vi "_fgv_debug.vi"(7 "Operation":T1=enum."ReadCommand", 8 "error in":errorcluster caption="error in (no error)", 9 "Command in":string, 11 "VISA resource name":refnum<visa-resource-name>) -> (0 "error out":errorcluster, 3 "VISA resource name out":refnum<visa-resource-name>)   [LabVIEW 2022 SP3, in "hmp4000_rsidr_core.lvlib"]
uses:
  hmp4000_rsidr_core.lvlib
  _type_Operation_Fgv_Debug.ctl
  type_Error_Codes.ctl
  Trim Whitespace One-Sided.vi
  Match Regular Expression.xnode
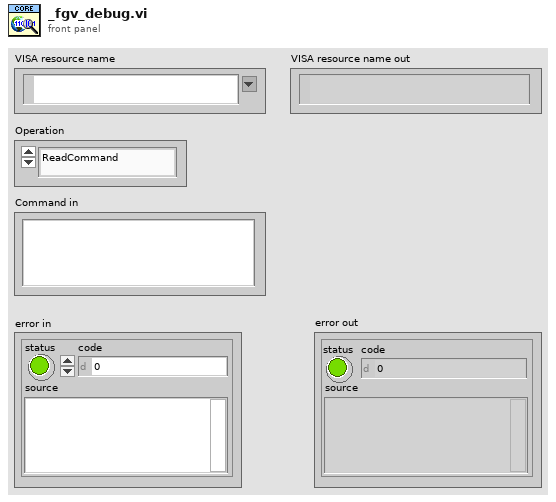
[diagram p1: front panel]
types:
  T1 = typedef "hmp4000_rsidr_core.lvlib/_type_Operation_Fgv_Debug.ctl" = enum16{"Reset", "ReadCommand", "SetCommand"}
  T2 = typedef "hmp4000_rsidr_core.lvlib/type_Error_Codes.ctl" = enum16{"No_error", "VISA_err_ResourceNotFound", "VISA_err_Timeout", "VISA_warn_MoreDataAvailable", "RS_err_MissingCallback", "RS_err_InvalidAttribute", "RS_err_InvalidValue", "RS_err_UnknownResource", "RS_err_AlreadyInitialized", "RS_err_InstrumentStatus", "RS_err_BadRepCapName", "RS_err_TypesMismatch", "RS_err_ValueNotSupported", "RS_err_InvalidRngTable", "RS_err_IDqueryFail", "RS_err_UnexpResponse", "VISA_warn_ConfigNotLoaded", "RS_err_AttributeNotReadable", "RS_err_AttributeNotWritable", "RS_err_InstrumentType", "RS_err_InstrumentOption", "VISA_err_InvalidSize", "RS_err_ReliabilityIndicator", "VISA_warn_UnknownStatus", "VISA_warn_TermCharRead", "VISA_err_IO_error", "RS_err_FunctionNotSupported", "VISA_warn_QueueEmpty"}
  T3 = typedef "hmp4000_rsidr_core.lvlib/type_Session_Data.ctl" = cluster{"IDN string":string, "Instrument FW":string, "Instr type":string, "Instr type for err. msg.":string, "Installed Options":string[], "Ignore Error Messages":string, "Logging params":variant, "OPC Timeout":i32, "VISA Timeout":i32, "STB Poll VISA Timeout":i32, "Additional Flags":i32, "Wait Before Read":i32, "Wait Before Write":i32, "Option String Flags":i32, "IO Segment Size":i64, "VISA Access Mode":T4, "Interface Type":T5, "OPC Wait Mode":T6, "Bin Float Number  Format":T7, "Bin Integer Number Format":T8, "Simulate":bool, "VXIcapable":bool, "Duplicate Session":bool, "Add LF to Write":bool, "Logging":bool, "Fast Sweep":bool, "Query Instrument Status":bool, "Check Range":bool, "Check Options":bool}
  T4 = typedef "hmp4000_rsidr_core.lvlib/type_VisaAccessMode.ctl" = u16
  T5 = typedef "hmp4000_rsidr_core.lvlib/type_InterfaceType.ctl" = enum16{"Unknown", "GPIB", "VXI", "GPIB_VXI", "ASRL", "PXI", "TCPIP", "USB", "SOCKET"}
  T6 = typedef "hmp4000_rsidr_core.lvlib/type_OPC_Wait_Mode.ctl" = enum16{"STBpolling", "STBpollingSlow", "STBpollingSuperSlow", "ServiceRequest", "OPCquery"}
  T7 = typedef "hmp4000_rsidr_core.lvlib/type_Binary_Float_Number_Format.ctl" = enum16{"Float_4_Bytes_Swapped", "Float_4_Bytes", "Double_8_Bytes_Swapped", "Double_8_Bytes"}
  T8 = typedef "hmp4000_rsidr_core.lvlib/type_Binary_Integer_Number_Format.ctl" = enum16{"Int32_4_Bytes_Swapped", "Int32_4 Bytes", "Int16_2_Bytes_Swapped", "Int16_2_Bytes"}
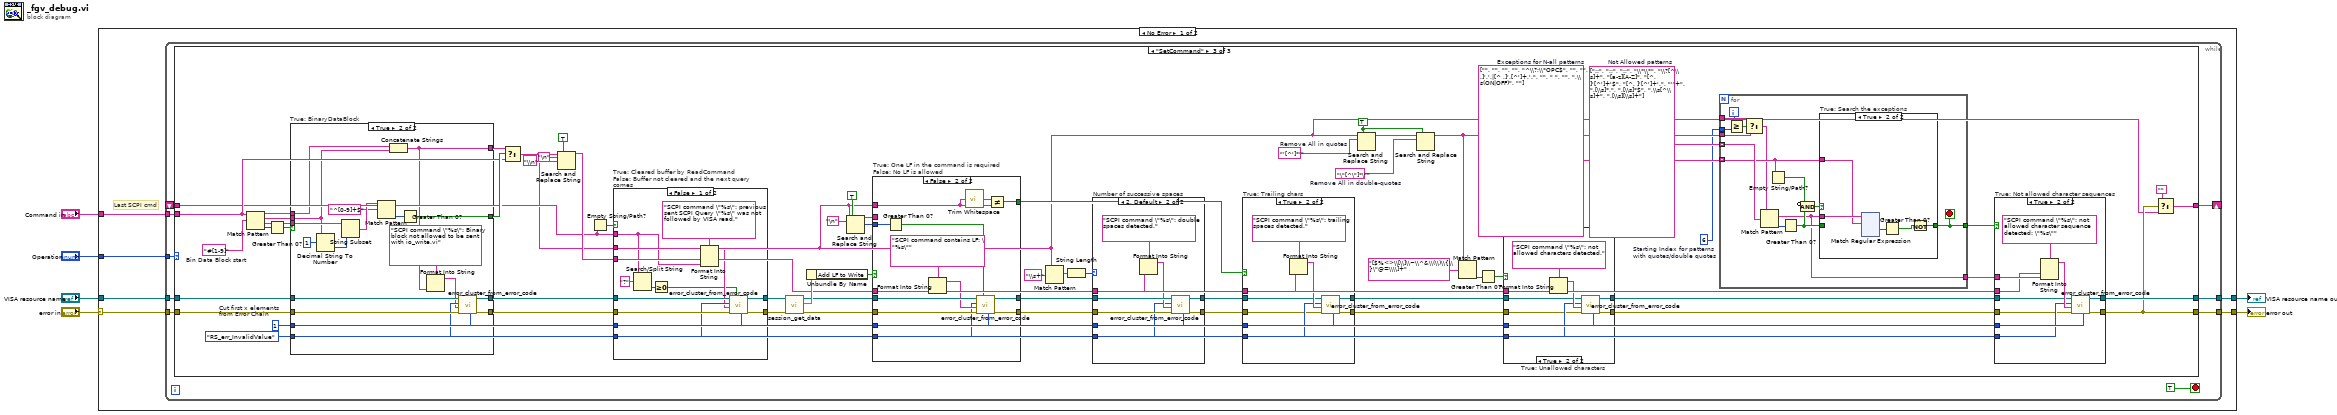
[diagram p0: block diagram]
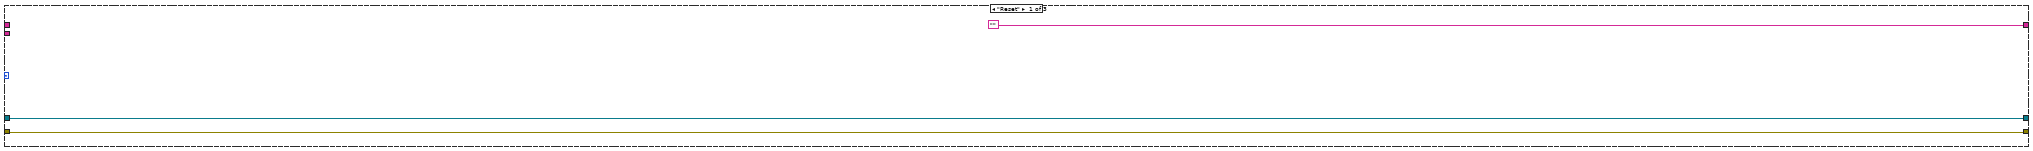
[diagram p2: hidden frame]
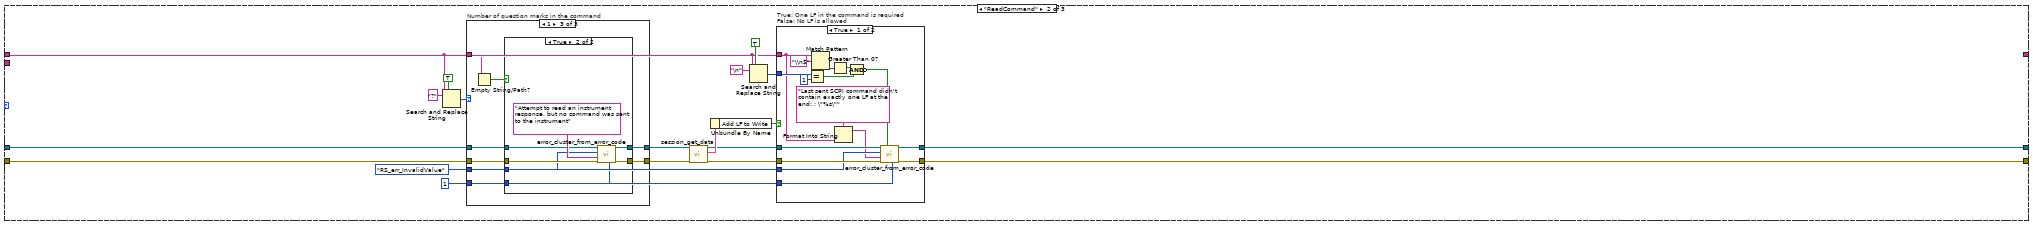
[diagram p3: hidden frame]
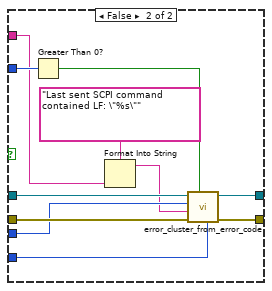
[diagram p4: hidden frame]
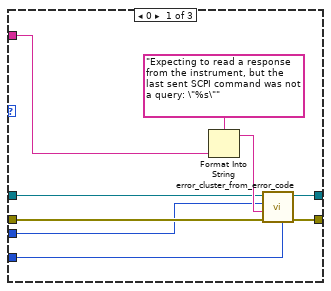
[diagram p5: hidden frame]
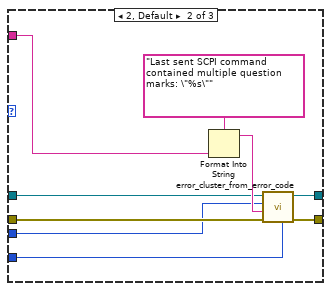
[diagram p6: hidden frame]
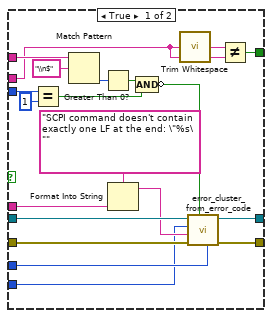
[diagram p13: hidden frame]
diagram:
  n1 = case shown="No Error" "error in" {
    selector: "error in" -> [w8 w420]
    tunnel: [w10 w420] -> w2
    tunnel: "Operation" -> [w12 _]
    tunnel: "Command in" -> [w11 _]
    tunnel: "VISA resource name" -> [w7 w419]
    tunnel: [w9 w419] -> w1
    frame No Error {
      # "Last SCPI cmd"
      n2 = while {
        shift-right: [w18] -> _
        shift-left: _ -> [w17]
        tunnel: w12 -> [w20]
        tunnel: w8 -> [w14]
        tunnel: w11 -> [w19]
        tunnel: w7 -> [w13]
        tunnel: [w16] -> w10
        tunnel: [w15] -> w9
        stop <- TRUE stop-if-true
        n3 = case shown="\"SetCommand\"" w20 {
          tunnel: w19 -> [_ _ w126]
          tunnel: ["" ("Empty String Constant") _ w161] -> w18
          tunnel: w17 -> [_ w28 w125]
          tunnel: w14 -> [w23 w40 w111]
          tunnel: w13 -> [w22 w39 w110]
          tunnel: [w23 w27 w140] -> w16
          tunnel: [w22 w26 w141] -> w15
          frame "Reset" {
          }
          frame "ReadCommand" {
            w25 = 1 ("Cut first x elements\nfrom Error Chain (0)")
            w31 = type_Error_Codes."RS_err_InvalidValue" ("Error Enum in")
            n4 = Search and Replace String(replace all?=TRUE ("replace all? (F)"), input string=w28, search string="?") -> (number of replacements=w41:i32)  [unwired: 5 in, 3 out]
            n5 = case "Number of question marks in the command" shown="1" w41 {
              tunnel: w40 -> [w78 w87 w94]
              tunnel: [w77 w86 w92] -> w38
              tunnel: w28 -> [w76 w85 w96]
              tunnel: w39 -> [w74 w82 w93]
              tunnel: [w73 w84 w91] -> w37
              tunnel: w31 -> [w72 w81 w90]
              tunnel: w25 -> [w71 w80 w89]
              frame 0 {
                n6 = Format Into String(format string="Expecting to read a response from the instrument, but the last sent SCPI command was not a query: \"%s\"", w76) -> (resulting string=w75:string)  [unwired: 2 in, 1 out]
                n7 = call "error_cluster_from_error_code.vi"("Cut first x elements\nfrom Error Chain (0)"=w71, "error in"=w78, "Error Message (\"\")"=w75, "Error Enum in"=w72, "VISA resource name"=w74) -> ("error out"=w77:errorcluster, "VISA resource name out"=w73:refnum<visa-resource-name>)  [unwired: 5 in]
              }
              frame 2, Default {
                n8 = Format Into String(format string="Last sent SCPI command contained multiple question marks: \"%s\"", w85) -> (resulting string=w83:string)  [unwired: 2 in, 1 out]
                n9 = call "error_cluster_from_error_code.vi"("Cut first x elements\nfrom Error Chain (0)"=w80, "error in"=w87, "Error Message (\"\")"=w83, "Error Enum in"=w81, "VISA resource name"=w82) -> ("error out"=w86:errorcluster, "VISA resource name out"=w84:refnum<visa-resource-name>)  [unwired: 5 in]
              }
              frame 1 {
                n10 = Empty String/Path?(string/path=w96) -> (empty?=w95:bool)
                n11 = case shown="True" w95 {
                  tunnel: w94 -> [w98 w104]
                  tunnel: [w98 w102] -> w92
                  tunnel: w93 -> [w97 w103]
                  tunnel: [w97 w101] -> w91
                  tunnel: w90 -> [_ w100]
                  tunnel: w89 -> [_ w99]
                  frame False {
                  }
                  frame True {
                    n12 = call "error_cluster_from_error_code.vi"("Cut first x elements\nfrom Error Chain (0)"=w99, "error in"=w104, "Error Message (\"\")"="Attempt to read an instrument response, but no command was sent to the instrument" ("error message (\"\")"), "Error Enum in"=w100, "VISA resource name"=w103) -> ("error out"=w102:errorcluster, "VISA resource name out"=w101:refnum<visa-resource-name>)  [unwired: 5 in]
                  }
                }
              }
            }
            n13 = call "session_get_data.vi"("error in"=w38, "VISA resource name"=w37) -> ("error out"=w33:errorcluster, "Session User Data out"=w34:T3, "VISA resource name out"=w32:refnum<visa-resource-name>)  [unwired: 6 in, 1 out]
            n14 = Unbundle By Name(w34) -> ("Add LF to Write"=w30:bool)
            n15 = Search and Replace String(replace all?=TRUE ("replace all? (F)"), input string=w28, search string="\n" ("Line Feed Constant")) -> (number of replacements=w29:i32)  [unwired: 5 in, 3 out]
            n16 = case "True: One LF in the command is required\nFalse: No LF is allowed" shown="True" w30 {
              tunnel: w33 -> [w59 w70]
              tunnel: w32 -> [w58 w69]
              tunnel: w31 -> [w57 w68]
              tunnel: w29 -> [w56 w65]
              tunnel: w28 -> [w46 w61]
              tunnel: [w49 w67] -> w27
              tunnel: [w48 w66] -> w26
              tunnel: w25 -> [w44 w60]
              frame True {
                n17 = Equal?(x=w56, y=1) -> (x = y?=w51:bool)
                n18 = Match Pattern(string=w46, regular expression="\\n$") -> (offset past match=w53:i32)  [unwired: 1 in, 3 out]
                n19 = Greater Than 0?(x=w53) -> (x > 0?=w52:bool)
                n20 = Format Into String(format string="Last sent SCPI command didn't contain exactly one LF at the end: : \"%s\"", w46) -> (resulting string=w45:string)  [unwired: 2 in, 1 out]
                n21 = Compound Arithmetic op=AND(w52, w51) -> (invert w50:bool)
                n22 = call "error_cluster_from_error_code.vi"("Cut first x elements\nfrom Error Chain (0)"=w44, "Error Creation Enabled (True)"=w50, "error in"=w59, "Error Message (\"\")"=w45, "Error Enum in"=w57, "VISA resource name"=w58) -> ("error out"=w49:errorcluster, "VISA resource name out"=w48:refnum<visa-resource-name>)  [unwired: 4 in]
              }
              frame False {
                n23 = Greater Than 0?(x=w65) -> (x > 0?=w64:bool)
                n24 = Format Into String(format string="Last sent SCPI command contained LF: \"%s\"", w61) -> (resulting string=w62:string)  [unwired: 2 in, 1 out]
                n25 = call "error_cluster_from_error_code.vi"("Cut first x elements\nfrom Error Chain (0)"=w60, "Error Creation Enabled (True)"=w64, "error in"=w70, "Error Message (\"\")"=w62, "Error Enum in"=w68, "VISA resource name"=w69) -> ("error out"=w67:errorcluster, "VISA resource name out"=w66:refnum<visa-resource-name>)  [unwired: 4 in]
              }
            }
          }
          frame "SetCommand" {
            w117 = 6  # Starting Index for patterns with quotes/double quotes
            w121 = "\"[^\"]*\""  # Remove All in double-quotes
            w113 = "#[1-9]"  # Bin Data Block start
            w131 = string[] ["", "", "", "", "^\\?;\\*OPC$", "", "", "[^ ,]','.|[^ ,]',[^']+,'.", "", " ", "", ",\\s(ON|OFF)", ""]  # Exceptions for N-all patterns
            w122 = TRUE ("replace all? (F)")
            w106 = "'[^']*'"  # Remove All in quotes
            w145 = string[] ["::", ";;", ":;", "\\*\\*", "\\?[^\\s]+", "[a-z][A-Z]", "[^, ]'[^']+'$", "[^, ]'[^']+'.", "''+", ",[\\s]*,", ",[\\s]*$", ",\\s[^\\s]+", ",[\\s][\\s]+"]  # Not Allowed patterns
            w112 = 1  # Cut first x elements from Error Chain
            w107 = type_Error_Codes."RS_err_InvalidValue" ("Error Enum in")
            n26 = Match Pattern(string=w126, regular expression=w113) -> (before substring=w114:string, match substring=w116:string, after substring=w128:string, offset past match=w130:i32)  [unwired: 1 in]
            n27 = Greater Than 0?(x=w130) -> (x > 0?=w129:bool)
            n28 = case "True: BinaryDataBlock" shown="True" w129 {
              selector: w129 -> [w169 _]
              tunnel: w128 -> [_ w186]
              tunnel: w116 -> [_ w179]
              tunnel: [w169 w181] -> w127
              tunnel: [_ w170] -> w115
              tunnel: w114 -> [_ w180]
              tunnel: w112 -> [_ w174]
              tunnel: w111 -> [w167 w178]
              tunnel: w110 -> [w168 w177]
              tunnel: [w167 w176] -> w109
              tunnel: [w168 w175] -> w108
              tunnel: w107 -> [_ w173]
              frame False {
              }
              frame True {
                n29 = Decimal String To Number(string=w179, offset=1) -> (number=w185:i32)  [unwired: 1 in, 1 out]
                n30 = String Subset(string=w186, length (rest)=w185) -> (substring=w184:string)  [unwired: 1 in]
                n31 = Match Pattern(string=w184, regular expression="^[0-9]+$") -> (offset past match=w182:i32)  [unwired: 1 in, 3 out]
                n32 = Concatenate Strings(w180, w179) -> (w170:string)
                n33 = Greater Than 0?(x=w182) -> (x > 0?=w181:bool)
                n34 = Format Into String(format string="SCPI command \"%s\": Binary block not allowed to be sent with io_write.vi", w170) -> (resulting string=w171:string)  [unwired: 2 in, 1 out]
                n35 = call "error_cluster_from_error_code.vi"("Cut first x elements\nfrom Error Chain (0)"=w174, "error in"=w178, "Error Message (\"\")"=w171, "Error Enum in"=w173, "VISA resource name"=w177) -> ("error out"=w176:errorcluster, "VISA resource name out"=w175:refnum<visa-resource-name>)  [unwired: 5 in]
              }
            }
            n36 = Select(t=w115, s=w127, f=w126) -> (s? t:f=w118:string)
            n37 = Search and Replace String(replace all?=TRUE ("replace all? (F)"), input string=w118, search string="\n" ("Line Feed Constant"), replace string="\\n" ("input string")) -> (result string=w132:string)  [unwired: 4 in, 3 out]
            n38 = Empty String/Path?(string/path=w125) -> (empty?=w162:bool)
            n39 = case "True: Cleared buffer by ReadCommand\nFalse: Buffer not cleared and the next query comes" shown="False" w162 {
              tunnel: w125 -> [w411 _]
              tunnel: w109 -> [w415 w418]
              tunnel: [w414 w418] -> w152
              tunnel: w118 -> [_ _]
              tunnel: w112 -> [w410 _]
              tunnel: w107 -> [w409 _]
              tunnel: w108 -> [w408 w417]
              tunnel: [w407 w417] -> w153
              tunnel: w132 -> [w404 _]
              frame False {
                n40 = Search/Split String(string=w411, search string/char (-)="?") -> (offset of match=w413:i32)  [unwired: 1 in, 2 out]
                n41 = Greater Or Equal To 0?(x=w413) -> (x >= 0?=w405:bool)
                n42 = Format Into String(format string="SCPI command \"%s\": previous sent SCPI Query \"%s\" was not followed by VISA read.", w404, w411) -> (resulting string=w406:string)  [unwired: 2 in, 1 out]
                n43 = call "error_cluster_from_error_code.vi"("Cut first x elements\nfrom Error Chain (0)"=w410, "Error Creation Enabled (True)"=w405, "error in"=w415, "Error Message (\"\")"=w406, "Error Enum in"=w409, "VISA resource name"=w408) -> ("error out"=w414:errorcluster, "VISA resource name out"=w407:refnum<visa-resource-name>)  [unwired: 4 in]
              }
              frame True {
              }
            }
            n44 = call "session_get_data.vi"("error in"=w152, "VISA resource name"=w153) -> ("error out"=w157:errorcluster, "Session User Data out"=w158:T3, "VISA resource name out"=w156:refnum<visa-resource-name>)  [unwired: 6 in, 1 out]
            n45 = Unbundle By Name(w158) -> ("Add LF to Write"=w155:bool)
            n46 = Search and Replace String(replace all?=TRUE ("replace all? (F)"), input string=w118, search string="\n" ("Line Feed Constant")) -> (result string=w120:string, number of replacements=w154:i32)  [unwired: 5 in, 2 out]
            n47 = case "True: One LF in the command is required\nFalse: No LF is allowed" shown="False" w155 {
              tunnel: w157 -> [w378 w392]
              tunnel: w156 -> [w377 w391]
              tunnel: w154 -> [w376 w388]
              tunnel: w118 -> [w366 w380]
              tunnel: [w369 w390] -> w150
              tunnel: [w368 w389] -> w151
              tunnel: w112 -> [w364 w384]
              tunnel: w107 -> [w363 w383]
              tunnel: w132 -> [w362 w382]
              tunnel: w120 -> [w360 _]
              tunnel: [w359 w379] -> w119
              frame True {
                n48 = Equal?(x=w376, y=1) -> (x = y?=w371:bool)
                n49 = Match Pattern(string=w366, regular expression="\\n$") -> (offset past match=w373:i32)  [unwired: 1 in, 3 out]
                n50 = Greater Than 0?(x=w373) -> (x > 0?=w372:bool)
                n51 = Format Into String(format string="SCPI command doesn't contain exactly one LF at the end: \"%s\"", w362) -> (resulting string=w365:string)  [unwired: 2 in, 1 out]
                n52 = Compound Arithmetic op=AND(w372, w371) -> (invert w370:bool)
                n53 = call "Trim Whitespace.vi"("string"=w360) -> ("trimmed string"=w361:string)  [unwired: 1 in]
                n54 = call "error_cluster_from_error_code.vi"("Cut first x elements\nfrom Error Chain (0)"=w364, "Error Creation Enabled (True)"=w370, "error in"=w378, "Error Message (\"\")"=w365, "Error Enum in"=w363, "VISA resource name"=w377) -> ("error out"=w369:errorcluster, "VISA resource name out"=w368:refnum<visa-resource-name>)  [unwired: 4 in]
                n55 = Not Equal?(x=w361, y=w360) -> (x != y?=w359:bool)
              }
              frame False {
                n56 = Greater Than 0?(x=w388) -> (x > 0?=w387:bool)
                n57 = Format Into String(format string="SCPI command contains LF: \"%s\"", w382) -> (resulting string=w385:string)  [unwired: 2 in, 1 out]
                n58 = call "Trim Whitespace.vi"("string"=w380) -> ("trimmed string"=w381:string)  [unwired: 1 in]
                n59 = call "error_cluster_from_error_code.vi"("Cut first x elements\nfrom Error Chain (0)"=w384, "Error Creation Enabled (True)"=w387, "error in"=w392, "Error Message (\"\")"=w385, "Error Enum in"=w383, "VISA resource name"=w391) -> ("error out"=w390:errorcluster, "VISA resource name out"=w389:refnum<visa-resource-name>)  [unwired: 4 in]
                n60 = Not Equal?(x=w381, y=w380) -> (x != y?=w379:bool)
              }
            }
            n61 = Match Pattern(string=w118, regular expression="\\s+") -> (match substring=w165:string)  [unwired: 1 in, 3 out]
            n62 = String Length(string=w165) -> (length=w166:i32)
            n63 = case "Number of successive spaces" shown="2, Default" w166 {
              tunnel: w150 -> [w394 w403]
              tunnel: [w394 w402] -> w139
              tunnel: w151 -> [w393 w400]
              tunnel: [w393 w399] -> w138
              tunnel: w112 -> [_ w397]
              tunnel: w107 -> [_ w396]
              tunnel: w132 -> [_ w395]
              frame 0, 1 {
              }
              frame 2, Default {
                n64 = Format Into String(format string="SCPI command \"%s\": double spaces detected.", w395) -> (resulting string=w398:string)  [unwired: 2 in, 1 out]
                n65 = call "error_cluster_from_error_code.vi"("Cut first x elements\nfrom Error Chain (0)"=w397, "error in"=w403, "Error Message (\"\")"=w398, "Error Enum in"=w396, "VISA resource name"=w400) -> ("error out"=w402:errorcluster, "VISA resource name out"=w399:refnum<visa-resource-name>)  [unwired: 5 in]
              }
            }
            n66 = case "True: Trailing chars" shown="True" w119 {
              tunnel: w139 -> [w189 w194]
              tunnel: [w189 w192] -> w137
              tunnel: w138 -> [w188 w193]
              tunnel: [w188 w191] -> w136
              tunnel: w112 -> [_ w196]
              tunnel: w107 -> [_ w195]
              tunnel: w132 -> [_ w190]
              frame False {
              }
              frame True {
                n67 = Format Into String(format string="SCPI command \"%s\": trailing spaces detected.", w190) -> (resulting string=w197:string)  [unwired: 2 in, 1 out]
                n68 = call "error_cluster_from_error_code.vi"("Cut first x elements\nfrom Error Chain (0)"=w196, "error in"=w194, "Error Message (\"\")"=w197, "Error Enum in"=w195, "VISA resource name"=w193) -> ("error out"=w192:errorcluster, "VISA resource name out"=w191:refnum<visa-resource-name>)  [unwired: 5 in]
              }
            }
            n69 = Search and Replace String(replace all?=w122, input string=w118, search string=w106) -> (result string=w123:string)  [unwired: 5 in, 3 out]
            n70 = Search and Replace String(replace all?=w122, input string=w123, search string=w121) -> (result string=w124:string)  [unwired: 5 in, 3 out]
            n71 = Match Pattern(string=w124, regular expression="[$%<>\\[\\]\\~\\^&\\(\\)\\{\\}\"@=\\\\]+") -> (offset past match=w147:i32)  [unwired: 1 in, 3 out]
            n72 = Greater Than 0?(x=w147) -> (x > 0?=w148:bool)
            n73 = case "True: Unallowed characters" shown="True" w148 {
              tunnel: w137 -> [w349 w354]
              tunnel: [w349 w352] -> w142
              tunnel: w136 -> [w348 w353]
              tunnel: [w348 w351] -> w146
              tunnel: w112 -> [_ w356]
              tunnel: w107 -> [_ w355]
              tunnel: w132 -> [_ w350]
              frame False {
              }
              frame True {
                n74 = Format Into String(format string="SCPI command \"%s\": not allowed characters detected.", w350) -> (resulting string=w357:string)  [unwired: 2 in, 1 out]
                n75 = call "error_cluster_from_error_code.vi"("Cut first x elements\nfrom Error Chain (0)"=w356, "error in"=w354, "Error Message (\"\")"=w357, "Error Enum in"=w355, "VISA resource name"=w353) -> ("error out"=w352:errorcluster, "VISA resource name out"=w351:refnum<visa-resource-name>)  [unwired: 5 in]
              }
            }
            n76 = for {
              tunnel: w145 -> [w212] mode=indexing
              tunnel: [w199] -> w144
              tunnel: [w207] -> w143
              tunnel: w124 -> [w202]
              tunnel: w131 -> [w206] mode=indexing
              tunnel: w118 -> [w205]
              tunnel: w117 -> [w201]
              i -> [w204]
              stop <- w199 stop-if-true
              n77 = Greater Or Equal?(x=w204, y=w201) -> (x >= y?=w203:bool)
              n78 = Select(t=w205, s=w203, f=w202) -> (s? t:f=w200:string)
              n79 = Match Pattern(string=w200, regular expression=w212) -> (match substring=w207:string, offset past match=w211:i32)  [unwired: 1 in, 2 out]
              n80 = Empty String/Path?(string/path=w206) -> (empty?=w210:bool)
              n81 = Greater Than 0?(x=w211) -> (x > 0?=w208:bool)
              n82 = Compound Arithmetic op=AND(invert w210, w208) -> (w209:bool)
              n83 = case "True: Search the exceptions" shown="True" w209 {
                tunnel: w208 -> [w213 _]
                tunnel: w207 -> [_ w217]
                tunnel: w206 -> [_ w214]
                tunnel: [w213 w218] -> w199
                frame False {
                }
                frame True {
                  n84 = xnode ("Match Regular Expression")("input string"=w217, "regular expression"=w214) -> ("offset past match"=w216:i32)  [unwired: 4 in, 4 out]
                  n85 = Greater Than 0?(x=w216) -> (x > 0?=w215:bool)
                  n86 = Not(x=w215) -> (.not. x?=w218:bool)
                }
              }
            }
            n87 = case "True: Not allowed character sequences" shown="True" w144 {
              tunnel: w142 -> [w337 w343]
              tunnel: [w337 w341] -> w140
              tunnel: w146 -> [w336 w342]
              tunnel: [w336 w340] -> w141
              tunnel: w112 -> [_ w345]
              tunnel: w107 -> [_ w344]
              tunnel: w143 -> [_ w339]
              tunnel: w132 -> [_ w338]
              frame False {
              }
              frame True {
                n88 = Format Into String(format string="SCPI command \"%s\": not allowed character sequence detected: \"%s\"", w338, w339) -> (resulting string=w346:string)  [unwired: 2 in, 1 out]
                n89 = call "error_cluster_from_error_code.vi"("Cut first x elements\nfrom Error Chain (0)"=w345, "error in"=w343, "Error Message (\"\")"=w346, "Error Enum in"=w344, "VISA resource name"=w342) -> ("error out"=w341:errorcluster, "VISA resource name out"=w340:refnum<visa-resource-name>)  [unwired: 5 in]
              }
            }
            n90 = Select(t="" ("Empty String Constant"), s=w140, f=w118) -> (s? t:f=w161:string)
          }
        }
      }
    }
    frame Error {
    }
  }
  "error out" <- w2
  "VISA resource name out" <- w1
